vi "SetControlDisabled.vi"(8 "error in (no error)":errorcluster, 9 "State (0=enabled)":u8=1, 10 "Control Label":string, 11 "CtlLookup In":T1) -> (0 "error out":errorcluster, 3 "CtlLookup Out":T1)   [LabVIEW 2020, in "CtlReferences_API.lvlib"]
doc: "Used to disable/enable a control.\nThis uses a numeric control rather than the labVIEW enum to save space.\n0= enabled\n1= disabled\n2= disabled and greyed out\nDefault is to disable"
uses:
  CtlReferences_API.lvlib
  CtlReferences/TypeDefs/CtlLookup.ctl
  CtlReferences/CtlReferences.lvclass
  CtlReferences/GetCtlRef.vi
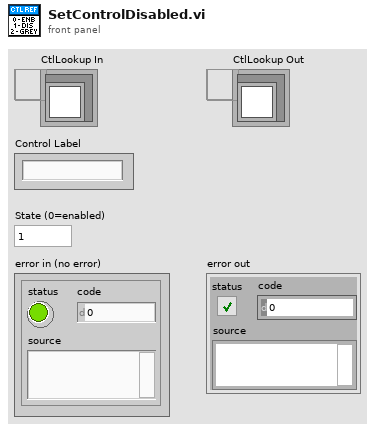
[diagram p1: front panel]
types:
  T1 = typedef "CtlReferences.lvlib/CtlReferences.lvclass/CtlLookup.ctl" = refnum<data-value>
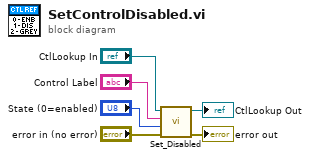
[diagram p0: block diagram]
diagram:
  n1 = call "Set_Disabled.vi"("error in (no error)"="error in (no error)", "State (0=enabled)"="State (0=enabled)", "Control Label"="Control Label", "CtlLookup In"="CtlLookup In") -> ("error out"=→"error out":errorcluster, "CtlLookup Out"=→"CtlLookup Out":T1)  [unwired: 6 in]
